vi "Executor.vi"(8 "error in (no error)":errorcluster, 9 "Semaphore":T1, 10 "Value":variant, 11 "Callbacks":refnum<queue>) -> ()   [LabVIEW 2017, in "Promise Future.lvlib" / "State.lvclass"]
uses:
  State.lvclass
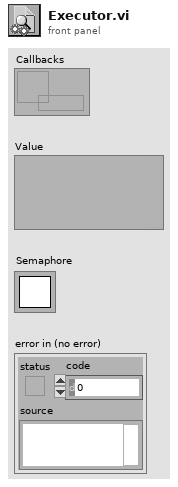
[diagram p1: front panel]
types:
  T1 = typedef "Semaphore RefNum" = refnum<k1>
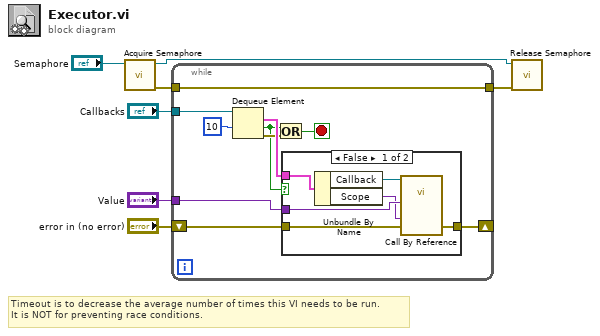
[diagram p0: block diagram]
diagram:
  # "Timeout is to decrease the average number of times this VI needs to be run.\nIt is NOT for preventing race conditions."
  n1 = call <vilib>:"Acquire Semaphore.vi"("semaphore"="Semaphore") -> ("error out"=w6:errorcluster, "semaphore out"=w5:T1)  [unwired: 4 in, 1 out]
  n2 = while {
    tunnel: "Callbacks" -> [w17]
    tunnel: "Value" -> [w16]
    tunnel: w6 -> [w10]
    tunnel: [w10] -> w7
    shift-right: [w9] -> _
    shift-left: "error in (no error)" -> [w14]
    stop <- w11 stop-if-true
    n3 = Dequeue Element(queue=w17, timeout in ms (-1)=10) -> (element=w15:cluster{"Callback":refnum<vi>, "Scope":variant}, timed out?=w12:bool, error out=w13:errorcluster)  [unwired: 1 in, 1 out]
    n4 = Or(x=w12, y=w13) -> (x .or. y?=w11:bool)
    n5 = case shown="False" w12 {
      tunnel: w16 -> [w23 _]
      tunnel: w15 -> [w20 _]
      tunnel: w14 -> [w22 w24]
      tunnel: [w21 w24] -> w9
      frame False {
        n6 = Unbundle By Name(w20) -> ("Callback"=w19:refnum<vi>, "Scope"=w18:variant)
        n7 = call-by-ref "?"(reference=w19, "error in (no error)"=w22, "Scope"=w18, "Value"=w23) -> ("error out"=w21:errorcluster)  [unwired: 9 in, 2 out]
      }
      frame True {
      }
    }
  }
  n8 = call <vilib>:"Release Semaphore.vi"("error in (no error)"=w7, "semaphore"=w5) -> ()  [unwired: 4 in, 2 out]
